vi "Walkabout.vi"(0 "reference in":refnum<class "Object.lvclass">, 5 "error in (no error)":errorcluster) -> (14 "reference out":refnum<class "Object.lvclass">, 19 "error out":errorcluster)   [LabVIEW 2020, in "Object.lvclass"]
doc: "This is the WalkAbout process that moves the object around the maze"
uses:
  Object.lvclass
  Map_class/Map.lvclass
  Map_class/SurfaceType.ctl
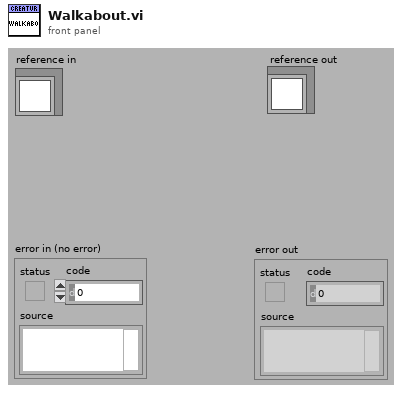
[diagram p1: front panel]
types:
  T1 = cluster{"Map":refnum<class "Map.lvclass">, "Tries":i32, "TriedStraight":bool}
  T2 = typedef "Map.lvclass/SurfaceType.ctl" = enum16{"Empty", "Wall"}
  T3 = typedef "Object.lvclass/ObjectAttributes.ctl" = cluster{"X":i32, "y":i32, "Heading":enum16{"N", "E", "S", "W"}, "Map":refnum<class "Map.lvclass">, "MovementDelay":i32, "Color":u32}
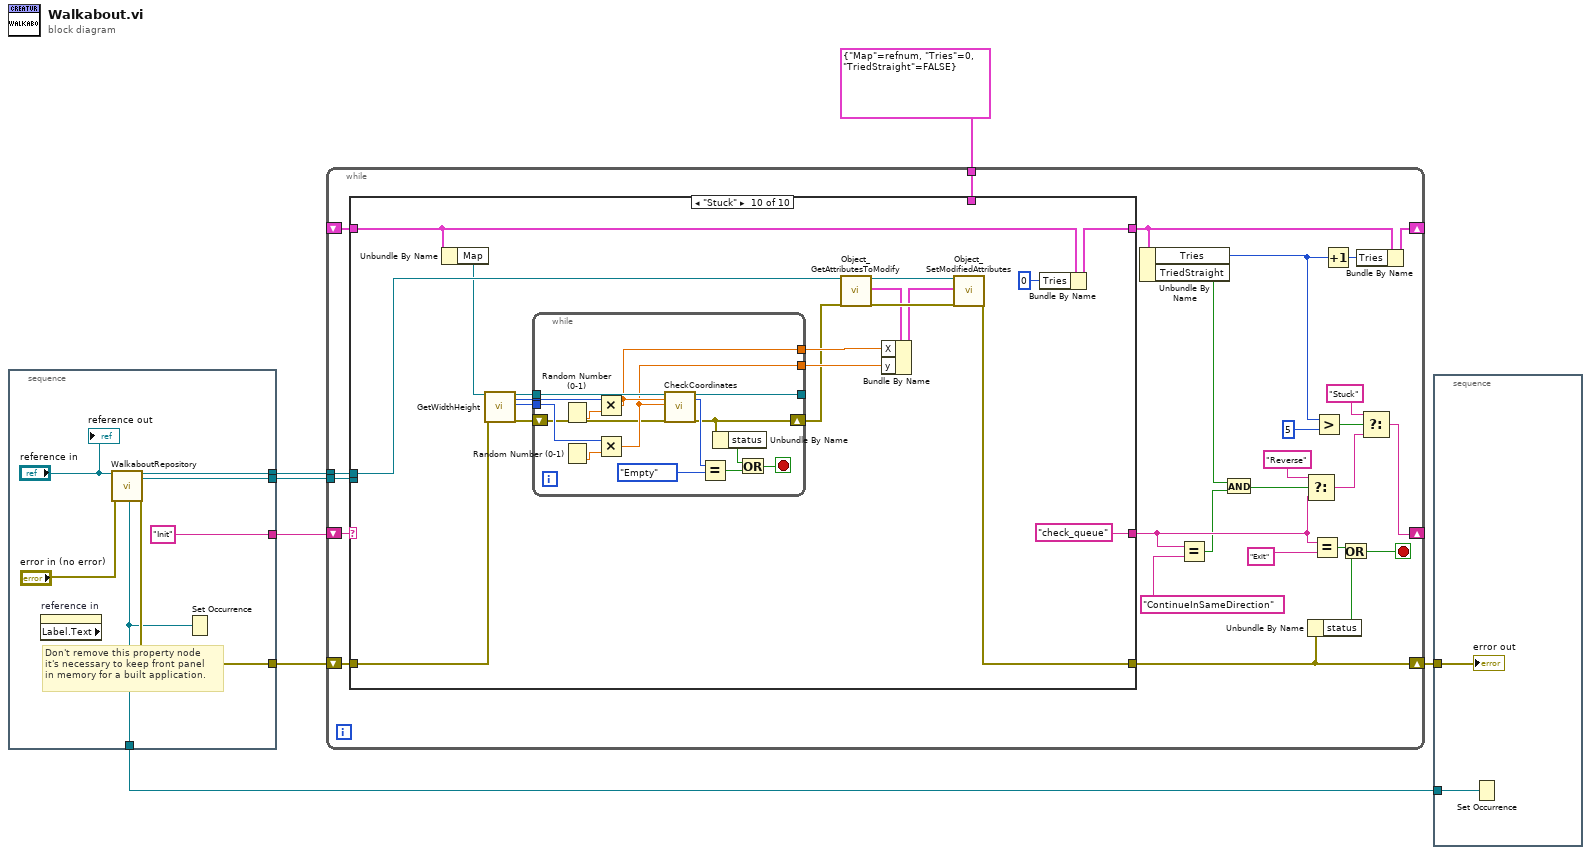
[diagram p0: block diagram]
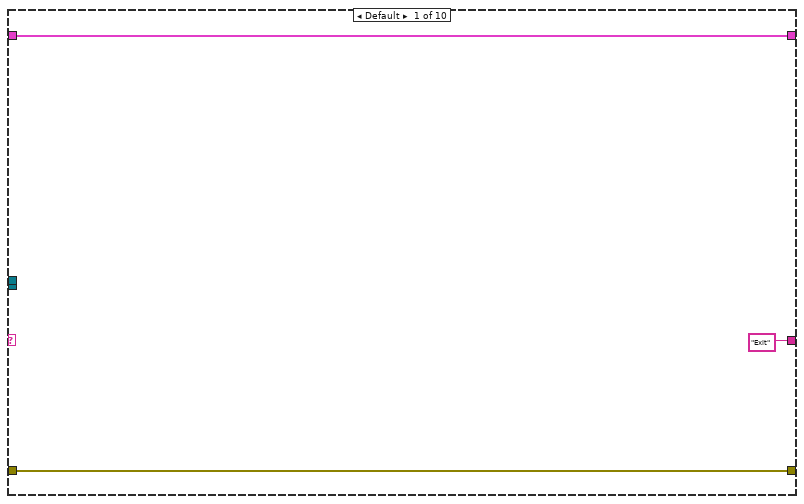
[diagram p2: hidden frame]
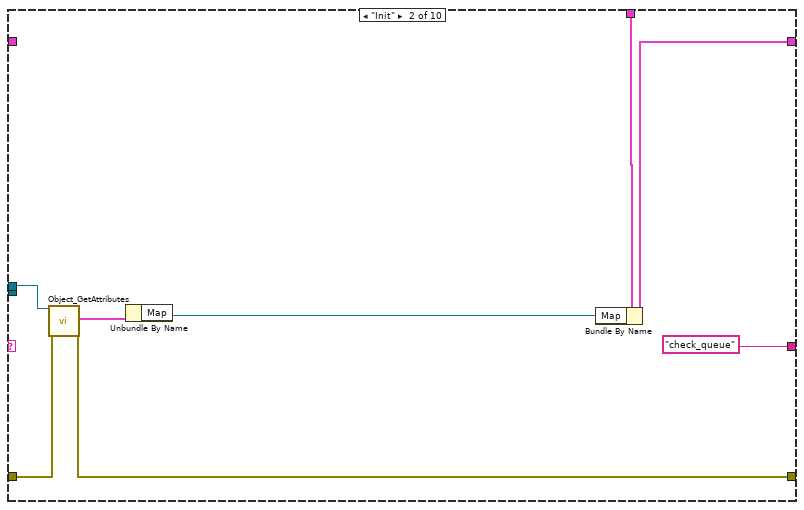
[diagram p3: hidden frame]
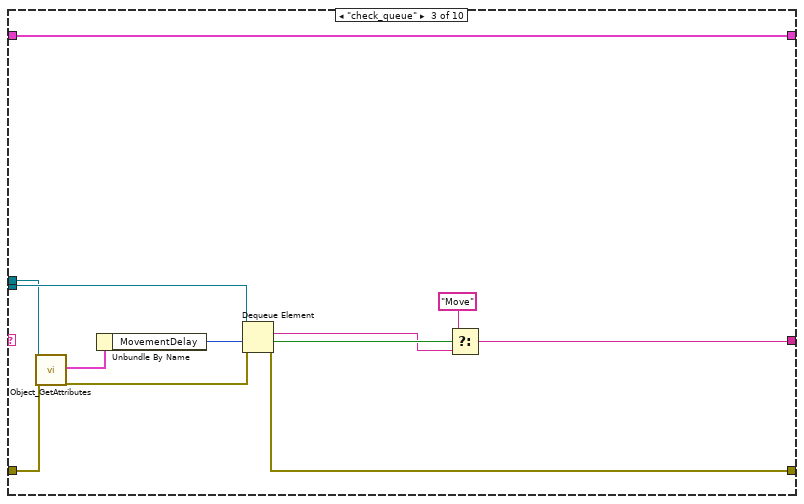
[diagram p4: hidden frame]
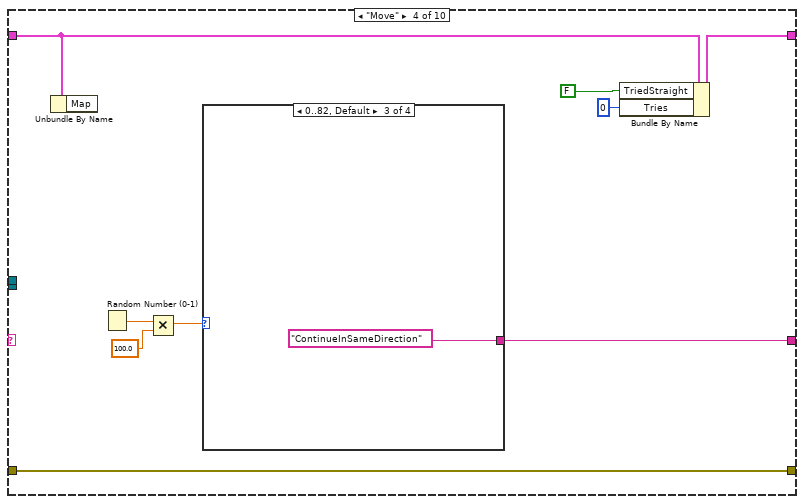
[diagram p5: hidden frame]
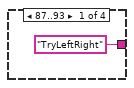
[diagram p6: hidden frame]
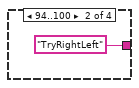
[diagram p7: hidden frame]
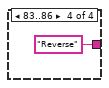
[diagram p8: hidden frame]
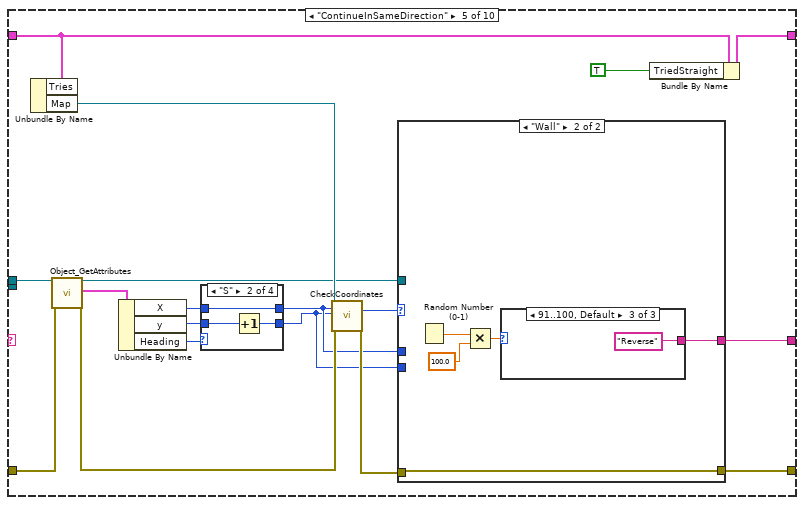
[diagram p9: hidden frame]
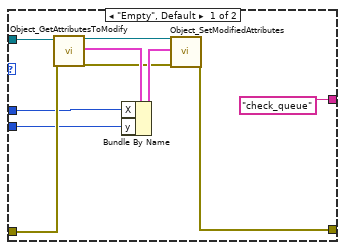
[diagram p10: hidden frame]
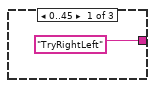
[diagram p11: hidden frame]
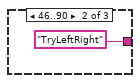
[diagram p12: hidden frame]
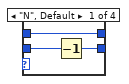
[diagram p13: hidden frame]
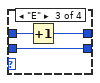
[diagram p14: hidden frame]
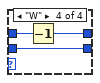
[diagram p15: hidden frame]
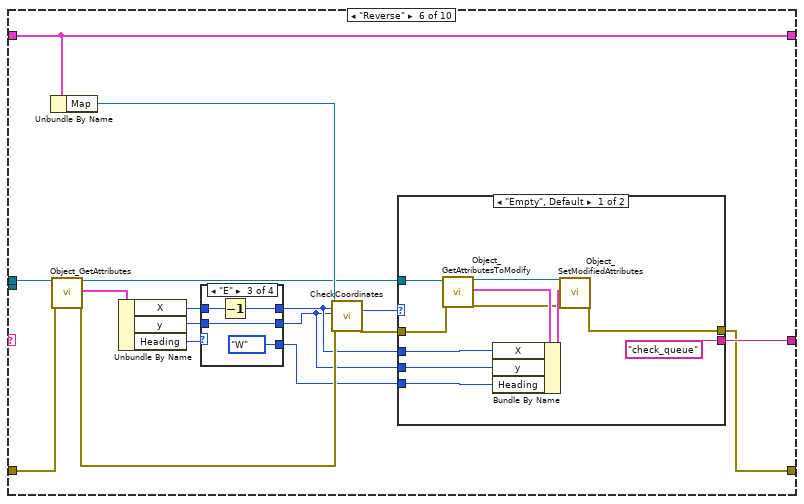
[diagram p16: hidden frame]
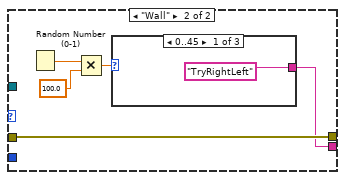
[diagram p17: hidden frame]
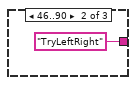
[diagram p18: hidden frame]
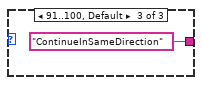
[diagram p19: hidden frame]
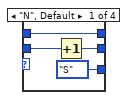
[diagram p20: hidden frame]
diagram:
  n1 = stacked-sequence {
    tunnel: [w11] -> w7
    tunnel: [w14] -> w5
    tunnel: [w10] -> w4
    tunnel: [w9] -> w3
    tunnel: ["Init"] -> w2
    frame #0 {
      # "Don't remove this property node\nit's necessary to keep front panel\nin memory for a built application."
      n2 = property on="reference in" class="LVClassControl (strict)" props=["Label", "Text"]() -> ()  [unwired: 2 in, 3 out]
      n3 = call "WalkaboutRepository.vi"("reference in"="reference in", "error in (no error)"="error in (no error)") -> ("ProcessSyncOccurrence"=w9:refnum<k4>, "reference out"=w14:refnum<class "Object.lvclass">, "ToProcessQueue"=w10:refnum<queue>, "error out"=w11:errorcluster)  [unwired: 14 out]
      n4 = Set Occurrence(w9) -> ()
      "reference out" <- "reference in"
    }
  }
  n5 = while {
    shift-right: [w37] -> w6
    shift-left: w7 -> [w38]
    tunnel: w5 -> [w39]
    tunnel: w4 -> [w40]
    shift-right: [w22] -> _
    shift-left: w2 -> [w34]
    shift-right: [w29] -> _
    shift-left: _ -> [w30]
    tunnel: T1 {"Map"=refnum, "Tries"=0, "TriedStraight"=FALSE} -> [w31]
    stop <- w35 stop-if-true
    n6 = case shown="\"Stuck\"" w34 {
      tunnel: w38 -> [w43 w49 w57 w70 w93 w139 w199 w294 w369 w374]
      tunnel: [w43 w45 w62 w70 w81 w126 w186 w283 w369 w373] -> w37
      tunnel: w40 -> [_ _ w63 _ _ _ _ _ _ _]
      tunnel: w39 -> [_ w50 w53 _ w87 w132 w192 w287 _ w377]
      tunnel: ["Exit" ("t") "check_queue" ("t") w58 w68 w80 w141 w200 w295 "Exit" ("t") "check_queue" ("t")] -> w19
      tunnel: w31 -> [_ w48 _ _ _ _ _ _ _ _]
      tunnel: [w42 w47 w52 w65 w78 w138 w198 w293 w367 w370] -> w28
      tunnel: w30 -> [w42 _ w52 w66 w79 w138 w198 w293 w367 w371]
      frame Default {
      }
      frame "Init" {
        n7 = call "Object_GetAttributes.vi"("reference in"=w50, "error in (no error)"=w49) -> ("Attributes"=w51:T3, "error out"=w45:errorcluster)  [unwired: 16 out]
        n8 = Unbundle By Name(w51) -> ("Map"=w46:refnum<class "Map.lvclass">)
        n9 = Bundle By Name(cluster=w48, "Map"=w46) -> (w47:T1)
      }
      frame "check_queue" {
        n10 = call "Object_GetAttributes.vi"("reference in"=w53, "error in (no error)"=w57) -> ("Attributes"=w56:T3, "error out"=w54:errorcluster)  [unwired: 16 out]
        n11 = Unbundle By Name(w56) -> ("MovementDelay"=w55:i32)
        n12 = Dequeue Element(queue=w63, timeout in ms (-1)=w55, error in (no error)=w54) -> (element=w60:string, timed out?=w61:bool, error out=w62:errorcluster)  [unwired: 1 out]
        n13 = Select(t="Move", s=w61, f=w60) -> (s? t:f=w58:string)
      }
      frame "Move" {
        n14 = Unbundle By Name(w66) -> ()  [unwired: 1 out]
        n15 = Random Number (0-1)() -> (number: 0 to 1=w72:dbl)
        n16 = Multiply(x=w72, y=100.0) -> (x*y=w69:dbl)
        n17 = case shown="0..82, Default" w69 {
          tunnel: ["TryLeftRight" ("t") "TryRightLeft" ("t") "ContinueInSameDirection" ("t") "Reverse" ("t")] -> w68
          frame 87..93 {
          }
          frame 94..100 {
          }
          frame 0..82, Default {
          }
          frame 83..86 {
          }
        }
        n18 = Bundle By Name(cluster=w66, "TriedStraight"=FALSE ("Can'tContinueStraight"), "Tries"=0) -> (w65:T1)
      }
      frame "ContinueInSameDirection" {
        n19 = Unbundle By Name(w79) -> ("Map"=w89:refnum<class "Map.lvclass">)  [unwired: 1 out]
        n20 = call "Object_GetAttributes.vi"("reference in"=w87, "error in (no error)"=w93) -> ("reference out"=w85:refnum<class "Object.lvclass">, "Attributes"=w94:T3, "error out"=w88:errorcluster)  [unwired: 15 out]
        n21 = Unbundle By Name(w94) -> ("X"=w90:i32, "y"=w91:i32, "Heading"=w92:enum16{"N", "E", "S", "W"})
        n22 = case shown="\"S\"" w92 {
          tunnel: w91 -> [w115 w118 w119 w122]
          tunnel: [w114 w117 w119 w122] -> w82
          tunnel: [w113 w116 w120 w123] -> w83
          tunnel: w90 -> [w113 w116 w121 w124]
          frame "N", Default {
            n23 = Decrement(x=w115) -> (x-1=w114:i32)
          }
          frame "S" {
            n24 = Increment(x=w118) -> (x+1=w117:i32)
          }
          frame "E" {
            n25 = Increment(x=w121) -> (x+1=w120:i32)
          }
          frame "W" {
            n26 = Decrement(x=w124) -> (x-1=w123:i32)
          }
        }
        n27 = call-dynamic "CheckCoordinates.vi"("reference in"=w89, "X"=w83, "Y"=w82, "error in (no error)"=w88) -> ("SurfaceType"=w86:T2, "error out"=w84:errorcluster)  [unwired: 14 out]
        n28 = case shown="\"Wall\"" w86 {
          tunnel: ["check_queue" ("t") w105] -> w80
          tunnel: w85 -> [w103 _]
          tunnel: w84 -> [w102 w109]
          tunnel: w83 -> [w98 _]
          tunnel: w82 -> [w97 _]
          tunnel: [w95 w109] -> w81
          frame "Empty", Default {
            n29 = call "Object_GetAttributesToModify.vi"("reference in"=w103, "error in (no error)"=w102) -> ("reference out"=w101:refnum<class "Object.lvclass">, "Attributes"=w100:T3, "error out"=w96:errorcluster)  [unwired: 1 in, 14 out]
            n30 = Bundle By Name(cluster=w100, "X"=w98, "y"=w97) -> (w99:T3)
            n31 = call "Object_SetModifiedAttributes.vi"("reference in"=w101, "Attributes"=w99, "error in (no error)"=w96) -> ("error out"=w95:errorcluster)  [unwired: 3 in, 13 out]
          }
          frame "Wall" {
            n32 = Random Number (0-1)() -> (number: 0 to 1=w108:dbl)
            n33 = Multiply(x=w108, y=100.0) -> (x*y=w106:dbl)
            n34 = case shown="91..100, Default" w106 {
              tunnel: ["TryRightLeft" ("t") "TryLeftRight" ("t") "Reverse" ("t")] -> w105
              frame 0..45 {
              }
              frame 46..90 {
              }
              frame 91..100, Default {
              }
            }
          }
        }
        n35 = Bundle By Name(cluster=w79, "TriedStraight"=TRUE ("Can'tContinueStraight")) -> (w78:T1)
      }
      frame "Reverse" {
        n36 = Unbundle By Name(w138) -> ("Map"=w134:refnum<class "Map.lvclass">)
        n37 = call "Object_GetAttributes.vi"("reference in"=w132, "error in (no error)"=w139) -> ("reference out"=w130:refnum<class "Object.lvclass">, "Attributes"=w140:T3, "error out"=w133:errorcluster)  [unwired: 15 out]
        n38 = Unbundle By Name(w140) -> ("X"=w135:i32, "y"=w136:i32, "Heading"=w137:enum16{"N", "E", "S", "W"})
        n39 = case shown="\"E\"" w137 {
          tunnel: w136 -> [w164 w168 w170 w174]
          tunnel: [w163 w167 w170 w174] -> w127
          tunnel: [w162 w166 w171 w175] -> w128
          tunnel: w135 -> [w162 w166 w172 w176]
          tunnel: [enum16{"N", "E", "S", "W"}."S" ("Heading") enum16{"N", "E", "S", "W"}."N" ("Heading") enum16{"N", "E", "S", "W"}."W" ("Heading") enum16{"N", "E", "S", "W"}."E" ("Heading")] -> w125
          frame "N", Default {
            n40 = Increment(x=w164) -> (x+1=w163:i32)
          }
          frame "S" {
            n41 = Decrement(x=w168) -> (x-1=w167:i32)
          }
          frame "E" {
            n42 = Decrement(x=w172) -> (x-1=w171:i32)
          }
          frame "W" {
            n43 = Increment(x=w176) -> (x+1=w175:i32)
          }
        }
        n44 = call-dynamic "CheckCoordinates.vi"("reference in"=w134, "X"=w128, "Y"=w127, "error in (no error)"=w133) -> ("SurfaceType"=w131:T2, "error out"=w129:errorcluster)  [unwired: 14 out]
        n45 = case shown="\"Empty\", Default" w131 {
          tunnel: ["check_queue" ("t") w153] -> w141
          tunnel: w130 -> [w151 _]
          tunnel: w129 -> [w150 w157]
          tunnel: w128 -> [w146 _]
          tunnel: w127 -> [w145 _]
          tunnel: [w143 w157] -> w126
          tunnel: w125 -> [w142 _]
          frame "Empty", Default {
            n46 = call "Object_GetAttributesToModify.vi"("reference in"=w151, "error in (no error)"=w150) -> ("reference out"=w149:refnum<class "Object.lvclass">, "Attributes"=w148:T3, "error out"=w144:errorcluster)  [unwired: 1 in, 14 out]
            n47 = Bundle By Name(cluster=w148, "X"=w146, "y"=w145, "Heading"=w142) -> (w147:T3)
            n48 = call "Object_SetModifiedAttributes.vi"("reference in"=w149, "Attributes"=w147, "error in (no error)"=w144) -> ("error out"=w143:errorcluster)  [unwired: 3 in, 13 out]
          }
          frame "Wall" {
            n49 = Random Number (0-1)() -> (number: 0 to 1=w156:dbl)
            n50 = Multiply(x=w156, y=100.0) -> (x*y=w154:dbl)
            n51 = case shown="0..45" w154 {
              tunnel: ["TryRightLeft" ("t") "TryLeftRight" ("t") "ContinueInSameDirection" ("t")] -> w153
              frame 0..45 {
              }
              frame 46..90 {
              }
              frame 91..100, Default {
              }
            }
          }
        }
      }
      frame "TryLeftRight" {
        # "Right"
        # "Left"
        n52 = call "Object_GetAttributes.vi"("reference in"=w192, "error in (no error)"=w199) -> ("reference out"=w190:refnum<class "Object.lvclass">, "Attributes"=w181:T3, "error out"=w193:errorcluster)  [unwired: 15 out]
        n53 = Unbundle By Name(w198) -> ("Map"=w194:refnum<class "Map.lvclass">)
        n54 = Unbundle By Name(w181) -> ("X"=w195:i32, "y"=w196:i32, "Heading"=w197:enum16{"N", "E", "S", "W"})
        n55 = Unbundle By Name(w181) -> ("X"=w184:i32, "y"=w183:i32, "Heading"=w182:enum16{"N", "E", "S", "W"})
        n56 = case shown="\"S\"" w197 {
          tunnel: w196 -> [w257 w261 w267 w271]
          tunnel: [w257 w261 w266 w270] -> w187
          tunnel: [w258 w262 w265 w269] -> w188
          tunnel: w195 -> [w259 w263 w265 w269]
          tunnel: [enum16{"N", "E", "S", "W"}."W" ("Heading") enum16{"N", "E", "S", "W"}."E" ("Heading") enum16{"N", "E", "S", "W"}."N" ("Heading") enum16{"N", "E", "S", "W"}."S" ("Heading")] -> w185
          frame "N", Default {
            n57 = Decrement(x=w259) -> (x-1=w258:i32)
          }
          frame "S" {
            n58 = Increment(x=w263) -> (x+1=w262:i32)
          }
          frame "E" {
            n59 = Decrement(x=w267) -> (x-1=w266:i32)
          }
          frame "W" {
            n60 = Increment(x=w271) -> (x+1=w270:i32)
          }
        }
        n61 = case shown="\"S\"" w182 {
          tunnel: w183 -> [w202 w206 w212 w216]
          tunnel: [w202 w206 w211 w215] -> w178
          tunnel: [w203 w207 w210 w214] -> w179
          tunnel: w184 -> [w204 w208 w210 w214]
          tunnel: [enum16{"N", "E", "S", "W"}."E" ("Heading") enum16{"N", "E", "S", "W"}."W" ("Heading") enum16{"N", "E", "S", "W"}."S" ("Heading") enum16{"N", "E", "S", "W"}."N" ("Heading")] -> w177
          frame "N", Default {
            n62 = Increment(x=w204) -> (x+1=w203:i32)
          }
          frame "S" {
            n63 = Decrement(x=w208) -> (x-1=w207:i32)
          }
          frame "E" {
            n64 = Increment(x=w212) -> (x+1=w211:i32)
          }
          frame "W" {
            n65 = Decrement(x=w216) -> (x-1=w215:i32)
          }
        }
        n66 = call-dynamic "CheckCoordinates.vi"("reference in"=w194, "X"=w188, "Y"=w187, "error in (no error)"=w193) -> ("reference out"=w180:refnum<class "Map.lvclass">, "SurfaceType"=w191:T2, "error out"=w189:errorcluster)  [unwired: 13 out]
        n67 = case shown="\"Wall\"" w191 {
          tunnel: ["check_queue" ("t") w237] -> w200
          tunnel: w190 -> [w226 w232]
          tunnel: w189 -> [w225 w236]
          tunnel: w188 -> [w221 _]
          tunnel: w187 -> [w220 _]
          tunnel: [w218 w231] -> w186
          tunnel: w185 -> [w217 _]
          tunnel: w180 -> [_ w235]
          tunnel: w179 -> [_ w230]
          tunnel: w178 -> [_ w229]
          tunnel: w177 -> [_ w228]
          frame "Empty", Default {
            n68 = call "Object_GetAttributesToModify.vi"("reference in"=w226, "error in (no error)"=w225) -> ("reference out"=w224:refnum<class "Object.lvclass">, "Attributes"=w223:T3, "error out"=w219:errorcluster)  [unwired: 1 in, 14 out]
            n69 = Bundle By Name(cluster=w223, "X"=w221, "y"=w220, "Heading"=w217) -> (w222:T3)
            n70 = call "Object_SetModifiedAttributes.vi"("reference in"=w224, "Attributes"=w222, "error in (no error)"=w219) -> ("error out"=w218:errorcluster)  [unwired: 3 in, 13 out]
          }
          frame "Wall" {
            n71 = call-dynamic "CheckCoordinates.vi"("reference in"=w235, "X"=w230, "Y"=w229, "error in (no error)"=w236) -> ("SurfaceType"=w234:T2, "error out"=w233:errorcluster)  [unwired: 14 out]
            n72 = case shown="\"Empty\", Default" w234 {
              tunnel: ["check_queue" ("t") w250] -> w237
              tunnel: w233 -> [w242 w249]
              tunnel: w232 -> [w243 _]
              tunnel: [w241 w249] -> w231
              tunnel: w230 -> [w240 _]
              tunnel: w229 -> [w239 _]
              tunnel: w228 -> [w238 _]
              frame "Empty", Default {
                n73 = call "Object_GetAttributesToModify.vi"("reference in"=w243, "error in (no error)"=w242) -> ("reference out"=w247:refnum<class "Object.lvclass">, "Attributes"=w246:T3, "error out"=w244:errorcluster)  [unwired: 1 in, 14 out]
                n74 = Bundle By Name(cluster=w246, "X"=w240, "y"=w239, "Heading"=w238) -> (w245:T3)
                n75 = call "Object_SetModifiedAttributes.vi"("reference in"=w247, "Attributes"=w245, "error in (no error)"=w244) -> ("error out"=w241:errorcluster)  [unwired: 3 in, 13 out]
              }
              frame "Wall" {
                n76 = Random Number (0-1)() -> (number: 0 to 1=w253:dbl)
                n77 = Multiply(x=w253, y=100.0) -> (x*y=w251:dbl)
                n78 = case shown="0..80" w251 {
                  tunnel: ["ContinueInSameDirection" ("t") "Reverse" ("t")] -> w250
                  frame 0..80 {
                  }
                  frame 81..100, Default {
                  }
                }
              }
            }
          }
        }
      }
      frame "TryRightLeft" {
        # "Right"
        # "Left"
        n79 = call "Object_GetAttributes.vi"("reference in"=w287, "error in (no error)"=w294) -> ("reference out"=w285:refnum<class "Object.lvclass">, "Attributes"=w279:T3, "error out"=w288:errorcluster)  [unwired: 15 out]
        n80 = Unbundle By Name(w293) -> ("Map"=w289:refnum<class "Map.lvclass">)
        n81 = Unbundle By Name(w279) -> ("X"=w290:i32, "y"=w291:i32, "Heading"=w292:enum16{"N", "E", "S", "W"})
        n82 = Unbundle By Name(w279) -> ("X"=w282:i32, "y"=w281:i32, "Heading"=w280:enum16{"N", "E", "S", "W"})
        n83 = case shown="\"W\"" w292 {
          tunnel: w291 -> [w352 w356 w362 w366]
          tunnel: [w352 w356 w361 w365] -> w273
          tunnel: [w353 w357 w360 w364] -> w274
          tunnel: w290 -> [w354 w358 w360 w364]
          tunnel: [enum16{"N", "E", "S", "W"}."W" ("Heading") enum16{"N", "E", "S", "W"}."E" ("Heading") enum16{"N", "E", "S", "W"}."N" ("Heading") enum16{"N", "E", "S", "W"}."S" ("Heading")] -> w272
          frame "N", Default {
            n84 = Decrement(x=w354) -> (x-1=w353:i32)
          }
          frame "S" {
            n85 = Increment(x=w358) -> (x+1=w357:i32)
          }
          frame "E" {
            n86 = Decrement(x=w362) -> (x-1=w361:i32)
          }
          frame "W" {
            n87 = Increment(x=w366) -> (x+1=w365:i32)
          }
        }
        n88 = case shown="\"E\"" w280 {
          tunnel: w281 -> [w297 w301 w307 w311]
          tunnel: [w297 w301 w306 w310] -> w275
          tunnel: [w298 w302 w305 w309] -> w276
          tunnel: w282 -> [w299 w303 w305 w309]
          tunnel: [enum16{"N", "E", "S", "W"}."E" ("Heading") enum16{"N", "E", "S", "W"}."W" ("Heading") enum16{"N", "E", "S", "W"}."S" ("Heading") enum16{"N", "E", "S", "W"}."N" ("Heading")] -> w277
          frame "N", Default {
            n89 = Increment(x=w299) -> (x+1=w298:i32)
          }
          frame "S" {
            n90 = Decrement(x=w303) -> (x-1=w302:i32)
          }
          frame "E" {
            n91 = Increment(x=w307) -> (x+1=w306:i32)
          }
          frame "W" {
            n92 = Decrement(x=w311) -> (x-1=w310:i32)
          }
        }
        n93 = call-dynamic "CheckCoordinates.vi"("reference in"=w289, "X"=w276, "Y"=w275, "error in (no error)"=w288) -> ("reference out"=w278:refnum<class "Map.lvclass">, "SurfaceType"=w286:T2, "error out"=w284:errorcluster)  [unwired: 13 out]
        n94 = case shown="\"Wall\"" w286 {
          tunnel: ["check_queue" ("t") w332] -> w295
          tunnel: w285 -> [w321 w327]
          tunnel: w284 -> [w320 w331]
          tunnel: [w315 w326] -> w283
          tunnel: w278 -> [_ w330]
          tunnel: w276 -> [w314 _]
          tunnel: w275 -> [w313 _]
          tunnel: w277 -> [w312 _]
          tunnel: w274 -> [_ w325]
          tunnel: w273 -> [_ w324]
          tunnel: w272 -> [_ w323]
          frame "Empty", Default {
            n95 = call "Object_GetAttributesToModify.vi"("reference in"=w321, "error in (no error)"=w320) -> ("reference out"=w319:refnum<class "Object.lvclass">, "Attributes"=w318:T3, "error out"=w316:errorcluster)  [unwired: 1 in, 14 out]
            n96 = Bundle By Name(cluster=w318, "X"=w314, "y"=w313, "Heading"=w312) -> (w317:T3)
            n97 = call "Object_SetModifiedAttributes.vi"("reference in"=w319, "Attributes"=w317, "error in (no error)"=w316) -> ("error out"=w315:errorcluster)  [unwired: 3 in, 13 out]
          }
          frame "Wall" {
            n98 = call-dynamic "CheckCoordinates.vi"("reference in"=w330, "X"=w325, "Y"=w324, "error in (no error)"=w331) -> ("SurfaceType"=w329:T2, "error out"=w328:errorcluster)  [unwired: 14 out]
            n99 = case shown="\"Empty\", Default" w329 {
              tunnel: ["check_queue" ("t") w345] -> w332
              tunnel: w328 -> [w337 w344]
              tunnel: w327 -> [w338 _]
              tunnel: [w336 w344] -> w326
              tunnel: w325 -> [w335 _]
              tunnel: w324 -> [w334 _]
              tunnel: w323 -> [w333 _]
              frame "Empty", Default {
                n100 = call "Object_GetAttributesToModify.vi"("reference in"=w338, "error in (no error)"=w337) -> ("reference out"=w342:refnum<class "Object.lvclass">, "Attributes"=w341:T3, "error out"=w339:errorcluster)  [unwired: 1 in, 14 out]
                n101 = Bundle By Name(cluster=w341, "X"=w335, "y"=w334, "Heading"=w333) -> (w340:T3)
                n102 = call "Object_SetModifiedAttributes.vi"("reference in"=w342, "Attributes"=w340, "error in (no error)"=w339) -> ("error out"=w336:errorcluster)  [unwired: 3 in, 13 out]
              }
              frame "Wall" {
                n103 = Random Number (0-1)() -> (number: 0 to 1=w348:dbl)
                n104 = Multiply(x=w348, y=100.0) -> (x*y=w346:dbl)
                n105 = case shown="81..100, Default" w346 {
                  tunnel: ["ContinueInSameDirection" ("t") "Reverse" ("t")] -> w345
                  frame 0..80 {
                  }
                  frame 81..100, Default {
                  }
                }
              }
            }
          }
        }
      }
      frame "shutdown" {
      }
      frame "Stuck" {
        n106 = Unbundle By Name(w371) -> ("Map"=w376:refnum<class "Map.lvclass">)
        n107 = call-dynamic "GetWidthHeight.vi"("reference in"=w376, "error in (no error)"=w374) -> ("reference out"=w381:refnum<class "Map.lvclass">, "Width"=w383:i32, "Height"=w382:i32, "error out"=w378:errorcluster)  [unwired: 14 out]
        n108 = while {
          tunnel: w383 -> [w403]
          tunnel: w382 -> [w400]
          tunnel: w381 -> [w399]
          tunnel: [w396] -> w380
          tunnel: [w395] -> w379
          tunnel: [w394] -> _
          shift-right: [w392] -> w375
          shift-left: w378 -> [w393]
          stop <- w389 stop-if-true
          n109 = Random Number (0-1)() -> (number: 0 to 1=w402:dbl)
          n110 = Random Number (0-1)() -> (number: 0 to 1=w401:dbl)
          n111 = Multiply(x=w403, y=w402) -> (x*y=w396:dbl)
          n112 = Multiply(x=w400, y=w401) -> (x*y=w395:dbl)
          n113 = call-dynamic "CheckCoordinates.vi"("reference in"=w399, "X"=w396, "Y"=w395, "error in (no error)"=w393) -> ("reference out"=w394:refnum<class "Map.lvclass">, "SurfaceType"=w398:T2, "error out"=w392:errorcluster)  [unwired: 13 out]
          n114 = Equal?(x=w398, y=SurfaceType."Empty") -> (x = y?=w391:bool)
          n115 = Unbundle By Name(w392) -> ("status"=w390:bool)
          n116 = Or(x=w390, y=w391) -> (x .or. y?=w389:bool)
        }
        n117 = call "Object_GetAttributesToModify.vi"("reference in"=w377, "error in (no error)"=w375) -> ("reference out"=w386:refnum<class "Object.lvclass">, "Attributes"=w385:T3, "error out"=w387:errorcluster)  [unwired: 1 in, 14 out]
        n118 = Bundle By Name(cluster=w385, "X"=w380, "y"=w379) -> (w384:T3)
        n119 = call "Object_SetModifiedAttributes.vi"("reference in"=w386, "Attributes"=w384, "error in (no error)"=w387) -> ("error out"=w373:errorcluster)  [unwired: 3 in, 13 out]
        n120 = Bundle By Name(cluster=w371, "Tries"=0) -> (w370:T1)
      }
    }
    n121 = Unbundle By Name(w28) -> ("Tries"=w23:i32, "TriedStraight"=w16:bool)
    n122 = Equal?(x=w19, y="ContinueInSameDirection" ("t")) -> (x = y?=w17:bool)
    n123 = And(x=w16, y=w17) -> (x .and. y?=w15:bool)
    n124 = Select(t="Reverse", s=w15, f=w19) -> (s? t:f=w21:string)
    n125 = Unbundle By Name(w37) -> ("status"=w36:bool)
    n126 = Equal?(x=w19, y="Exit" ("t")) -> (x = y?=w32:bool)
    n127 = Greater?(x=w23, y=5) -> (0:w25:bool)
    n128 = Increment(x=w23) -> (x+1=w27:i32)
    n129 = Or(x=w32, y=w36) -> (x .or. y?=w35:bool)
    n130 = Bundle By Name(cluster=w28, "Tries"=w27) -> (w29:T1)
    n131 = Select(t="Stuck", s=w25, f=w21) -> (s? t:f=w22:string)
  }
  n132 = stacked-sequence {
    tunnel: w6 -> [w405]
    tunnel: w3 -> [w404]
    frame #0 {
      n133 = Set Occurrence(w404) -> ()
      "error out" <- w405
    }
  }
